vi "test_init_and_run.vi"() -> ()   [LabVIEW 2015]
uses:
  fieldpoint_rw.lvclass
panel:
  out "Protocol_Generic out":refnum<class "fieldpoint_rw.lvclass">
  out "error out":errorcluster
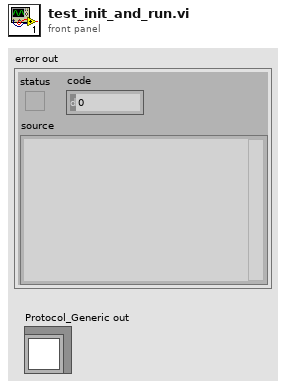
[diagram p1: front panel]
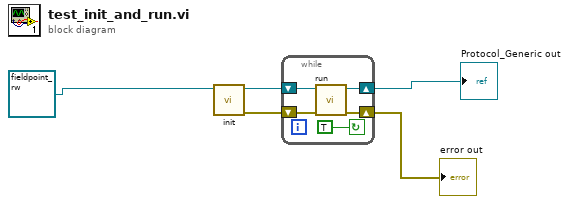
[diagram p0: block diagram]
diagram:
  n1 = call-dynamic "init.vi"("canon_m3 in"=refnum<class "fieldpoint_rw.lvclass"> refnum ("canon_m3.lvclass")) -> ("error out"=w4:errorcluster, "canon_m3 out"=w5:refnum<class "fieldpoint_rw.lvclass">)  [unwired: 9 in]
  n2 = while {
    shift-right: [w7] -> w2
    shift-left: w5 -> [w10]
    shift-right: [w8] -> w3
    shift-left: w4 -> [w9]
    stop <- TRUE continue-if-true
    n3 = call-dynamic "run.vi"("error in (no error)"=w9, "canon_m3 in"=w10) -> ("error out"=w8:errorcluster, "canon_m3 out"=w7:refnum<class "fieldpoint_rw.lvclass">)  [unwired: 8 in]
  }
  "error out" <- w3
  "Protocol_Generic out" <- w2
